vi "svfa_Initial Guess for Tone Estimation.vi"   [LabVIEW 2017]
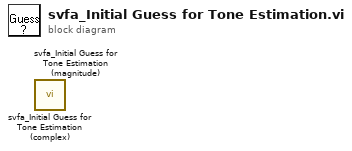
[diagram p0: block diagram]
diagram:
  n1 = call <vilib>:"svfa_Initial Guess for Tone Estimation (complex).vi"() -> ()  [unwired: 10 in, 2 out]
  n2 = call <vilib>:"svfa_Initial Guess for Tone Estimation (magnitude).vi"() -> ()  [unwired: 10 in, 2 out]
